vi "ProcessData.vi"(8 "error in (no error)":errorcluster, 9 "State":T1, 10 "Analog Data":T3, 11 "PassiveExperiment in":refnum<class "PassiveExperiment.lvclass">) -> (0 "error out":errorcluster, 1 "Fixated":bool, 2 "Trigger":T2=enum."Broke Fixation", 3 "PassiveExperiment out":refnum<class "PassiveExperiment.lvclass">)   [LabVIEW 2014, in "AcquisitionCoreObjects.lvlib" / "PassiveExperiment.lvclass"]
uses:
  PassiveExperiment.lvclass
  Core SubVIs/Controls/TYPE - Analog Data.ctl
  Trial Based Experiment.lvsc/Trigger.ctl
  Trial Based Experiment.lvsc/State.ctl
  <vilib>/measure/madcrms.llb/Basic Averaged DC-RMS for 1 Chan.vi
  Core SubVIs/Core SubVIs.lvlib
  <vilib>/measure/NI_MAPro.lvlib
  Trial Based Experiment.lvsc
  Acquisition/BehaviorData/BehaviorData.lvclass
panel:
  in  "Break Timeout (ms)":dbl
  in  "Adjustment Rate":dbl=0.02
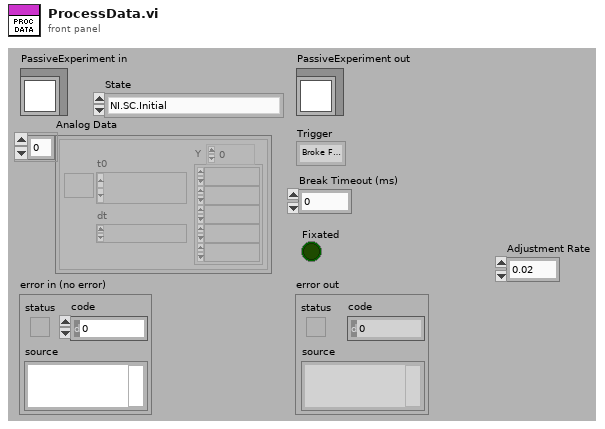
[diagram p1: front panel]
types:
  T1 = typedef "Trial Based Experiment.lvsc/State.ctl" = enum16{"NI.SC.Initial", "NI.SC.History", "NI.SC.ShallowHistory", "NI.SC.Terminal", "Cleanup", "State", "State\\Region\\Pause", "State\\Region\\Response Period", "State\\Region\\Delay Period", "State\\Region\\Hold Fixation", "State\\Region\\Acquire Fixation", "State\\Region\\Abort Trial", "State\\Region\\End Trial", "State\\Region\\Intertrial", "State\\Region\\Start Trial"}
  T2 = typedef "Trial Based Experiment.lvsc/Trigger.ctl" = enum16{"NULL", "Fixated", "Broke Fixation", "Stop", "Correct Response", "Incorrect Response", "Timeout"}
  T3 = typedef "Core SubVIs.lvlib/TYPE - Analog Data.ctl" = waveform(dbl)[]
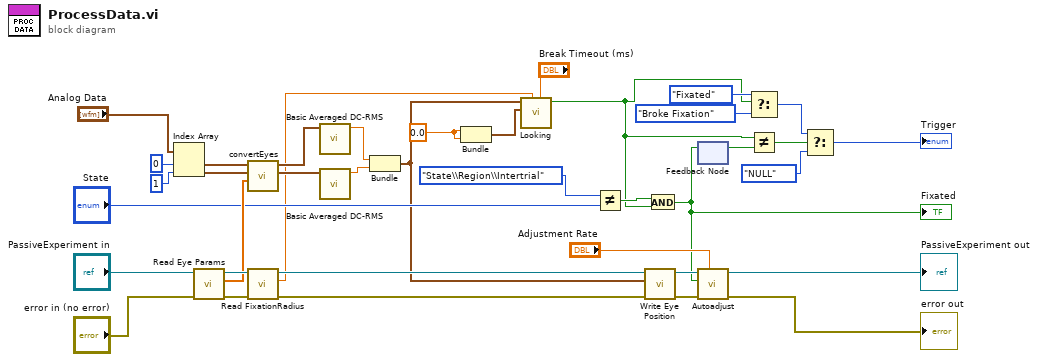
[diagram p0: block diagram]
diagram:
  w6 = 0.0
  n1 = Index Array(array="Analog Data", index #1=0 ("index"), index #2=1 ("index")) -> (element #1=w31:waveform(dbl), element #2=w30:waveform(dbl))
  n2 = call-dynamic "Read Eye Params.vi"("error in (no error)"="error in (no error)", "TrialBasedExperiment in"="PassiveExperiment in") -> ("error out"=w24:errorcluster, "Eye Params"=w32:dbl[], "TrialBasedExperiment out"=w38:refnum<class "PassiveExperiment.lvclass">)  [unwired: 7 in]
  n3 = call "convertEyes.vi"("Params"=w32, "Vertical"=w30, "Horizontal"=w31) -> ("Vertical Calibrated"=w35:waveform(dbl), "Horizontal Calibrated"=w34:waveform(dbl))  [unwired: 7 in]
  n4 = call-dynamic "Read FixationRadius.vi"("error in (no error)"=w24, "MatlabExperiment in"=w38) -> ("error out"=w18:errorcluster, "FixationRadius"=w3:dbl, "MatlabExperiment out"=w21:refnum<class "PassiveExperiment.lvclass">)  [unwired: 7 in]
  n5 = call-poly <vilib>:"Basic Averaged DC-RMS.vi"("signal in"=w34) -> ("DC value"=w23:dbl)  [unwired: 7 in, 3 out]
  n6 = call-poly <vilib>:"Basic Averaged DC-RMS.vi"("signal in"=w35) -> ("DC value"=w22:dbl)  [unwired: 7 in, 3 out]
  n7 = Bundle("DC value"=w23, "DC value"=w22) -> (w7:cluster{"DC value":dbl, "DC value":dbl})  [unwired: 1 in]
  n8 = Bundle(w6, w6) -> (w5:cluster{dbl, dbl})  [unwired: 1 in]
  n9 = call "Looking.vi"("Break Timeout (ms)"="Break Timeout (ms)", "Fixation Radius (px)"=w3, "Desired Position"=w5, "Eye Position"=w7) -> ("Looking"=w4:bool)  [unwired: 6 in, 1 out]
  n10 = Not Equal?(x=State."State\\Region\\Intertrial", y="State") -> (x != y?=w15:bool)
  n11 = call-dynamic "Write Eye Position.vi"("error in (no error)"=w18, "Eye Position"=w7, "TrialBasedExperiment in"=w21) -> ("error out"=w17:errorcluster, "TrialBasedExperiment out"=w20:refnum<class "PassiveExperiment.lvclass">)  [unwired: 7 in]
  n12 = And(x=w15, y=w4) -> (x .and. y?=w10:bool)
  "Fixated" <- w10
  n13 = feedback #1() -> (w27:bool)  [unwired: 1 in]
  n14 = feedback-in #1(w10) -> ()
  n15 = call-dynamic "Autoadjust.vi"("Adjustment Rate"="Adjustment Rate", "error in (no error)"=w17, "Fixated"=w10, "TrialBasedExperiment in"=w20) -> ("error out"=→"error out":errorcluster, "TrialBasedExperiment out"=→"PassiveExperiment out":refnum<class "PassiveExperiment.lvclass">)  [unwired: 6 in]
  n16 = Select(t=Trigger."Fixated" ("Trigger"), s=w4, f=Trigger."Broke Fixation" ("Trigger")) -> (s? t:f=w28:T2)
  n17 = Not Equal?(x=w4, y=w27) -> (x != y?=w25:bool)
  n18 = Select(t=w28, s=w25, f=Trigger."NULL" ("Trigger")) -> (s? t:f=→"Trigger":T2)
